vi "Симулятор 1553 windows.vi"() -> ()   [LabVIEW 2015]
panel:
  in  "Управление \nамплитудой, В":dbl(knob)=18.0 min=18.0 max=27.0 scale=18.0..27.0
  out "осталось слов для передачи":u8=1
  out "Режимы машины состояний ОУ":T1=enum."ожидание rising"
  out "Машина состояний КШ":T2
  out "Осталось принять слов":u8=1
  out "Принимаемые\nданные":u16[](array[numeric]) format="%04x"
  out "Передача?":bool=TRUE
  out "Ошибка \nпередачи на ОУ":bool
  out "Подадрес":u32
  out "Передача данных\n на ОУ?":bool
  out "Кол-во СД":u8
  in  "адрес этого\nОУ (0-30)":u8=8
  out "записаны данные":dbl
  out "Waveform Chart":T3(graph)
  out "счетчик длительн бита":u32
  out "T-F crossing":bool
  out "F-T crossing":bool
  in  "Кол-во слов \nдля приема":u8=4
  out "Ошибка \nчтения из ОУ":bool
  in  "RX":bool
  out "TX":bool
  in  "Команда управления":T4(ring)=enum."Блокировать передатчик"
  in  "Отправить команду ОУ":bool
  out "Данные при-\nнятые от КШ":u16[](array[numeric]) format="%04x"
  in  "Данные для\nотправки на КШ":u16[](array[numeric])=[12, 9, 11, 4, 5, 6, 7, 8, 9, 10, 11, 12, 13, 14, 15, 16, 17, 18, 19, 20, 21, 22, 23, 24, 25, 26, 27, 28, 29, 30, 31, 32] format="%04x"
  in  "Отправить\nTx CMD":bool
  in  "Отправить\nRx CMD":bool
  in  "Кол-во слов \nдля передачи":u8=3
  in  "Подадрес (1-30)":u8=1
  in  "адрес ОУ (0-30)":u8=8
  in  "Передаваемые данные":u16[](array[numeric])=[4, 821, 65535, 13380, 0, 0, 0, 0, 0, 0, 0, 0, 0, 0, 0, 0, 0, 0, 0, 0, 0, 0, 0, 0, 0, 0, 0, 0, 0, 0, 0, 0, 0, 0] format="%04x"
  # "Тестовая панель контроллера шины  MIL STD 1553"
  # "Настройки"
  # "Команда передачи:"
  # "Управление ОУ:"
  # "Команда чтения:"
  # "Тестовая панель оконечного устройства шины  MIL STD 1553"
  # "Прием КС:"
  # "Получение:"
  # "Передача:"
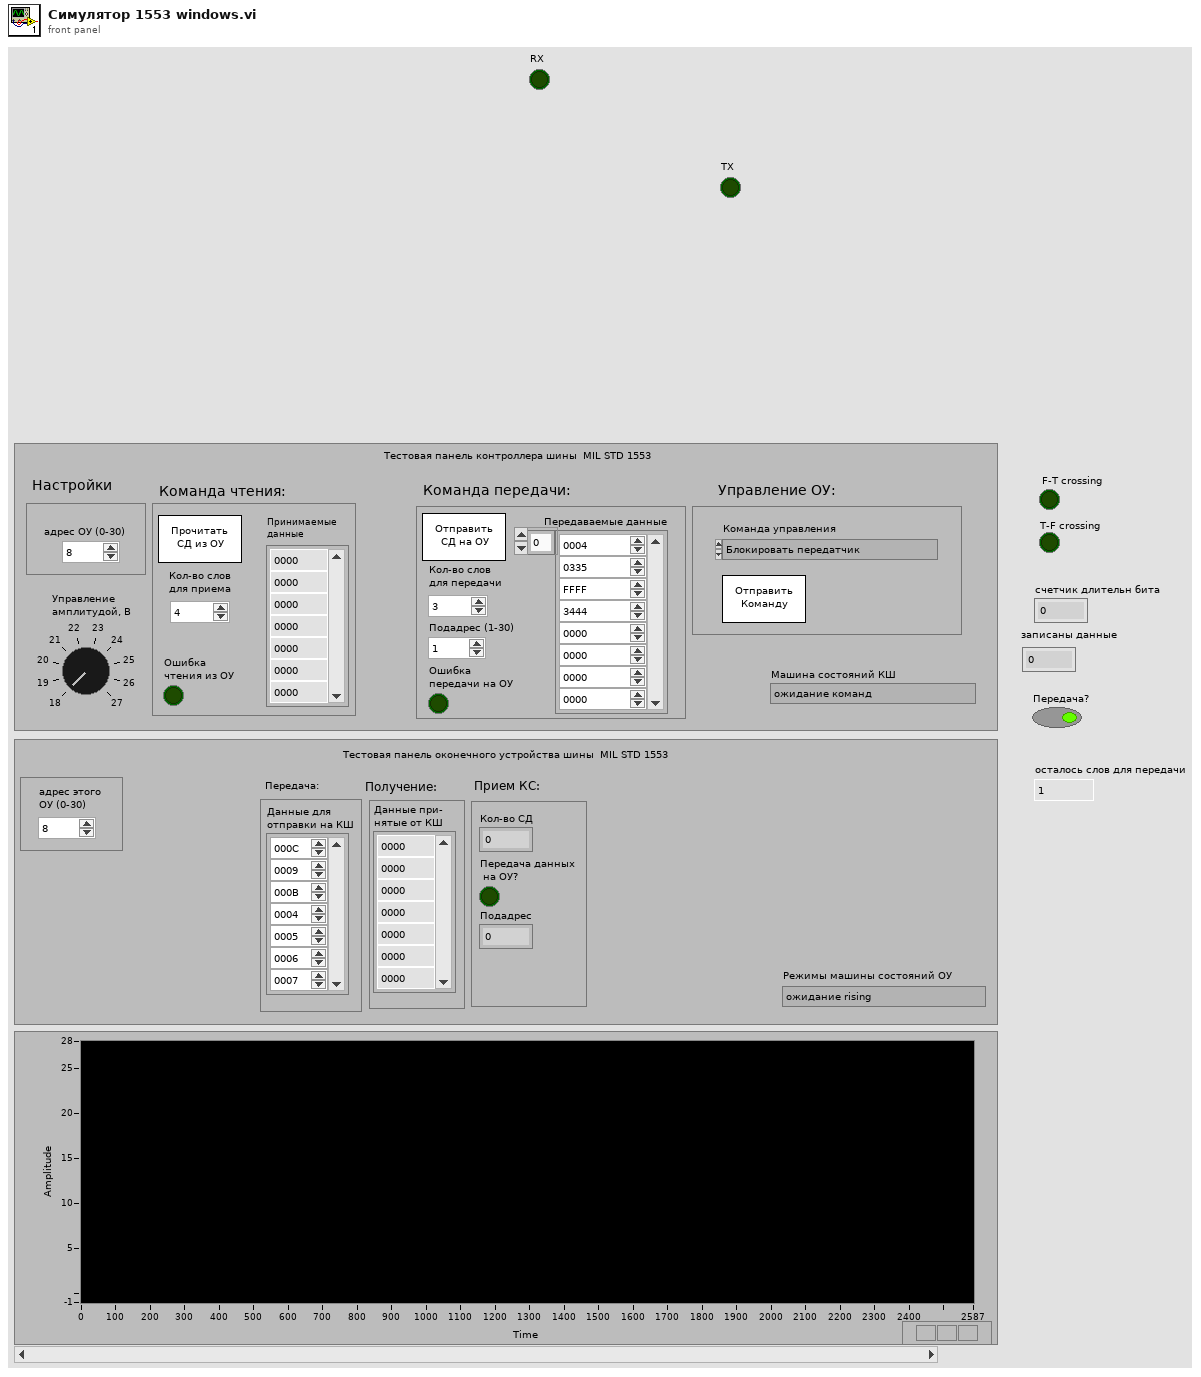
[diagram p1: front panel]
types:
  T1 = typedef "машина состояний ОУ.ctl" = enum16{"замер длительности true", "отправка СД", "кодирование СД", "ожидание rising", "ожидание rising СД", "чтение СД", "чтение КС", "замер длительности true СД", "замер длительности false", "чтение бит КС", "манчестер декодер СД", "манчестер декодер", "чтение бит СД", "подготовка ОС", "кодирование ОС", "отправка ОС", "подготовка СД"}
  T2 = typedef "машина состояний КШ.ctl" = enum16{"ожидание команд", "Подготовка команды RX", "Подготовка команды TX", "кодер манчестер КС", "таймаут t2 между словами", "Передача", "ожидание rising СД", "замер длительности true СД", "чтение бит СД", "манчестер декодер СД", "чтение СД", "ожидание rising ОС", "замер длительности false ОС", "замер длительности true OC", "чтение бит ОС", "манчестер декодер ОС", "чтение ОС", "подготовка СД", "кодирование СД", "отправка СД"}
  T3 = cluster{i16, dbl, "f":dbl, dbl, "записаны данные":dbl}
  T4 = enum16{"Принять управление интерфейсом", "Синхронизация", "Передать ОС", "Начать самоконтроль ОУ", "Блокировать передатчик", "Разблокировать передатчик", "Блокировать признак неисправности ОУ", "Разблокировать признак неисправнотси ОУ", "Установить ОУ в исходное состояние", "Резерв", "Передать векорное слово", "Синхронизвция с СД", "Передать последнюю команду", "Передать слово ВСК ОУ", "Блокировать i-й передатчик", "Разблокировать i-й передатчик", "Резерв 2"}
  T5 = cluster{i16, "f":dbl, "f":dbl, dbl, "записаны данные":dbl}
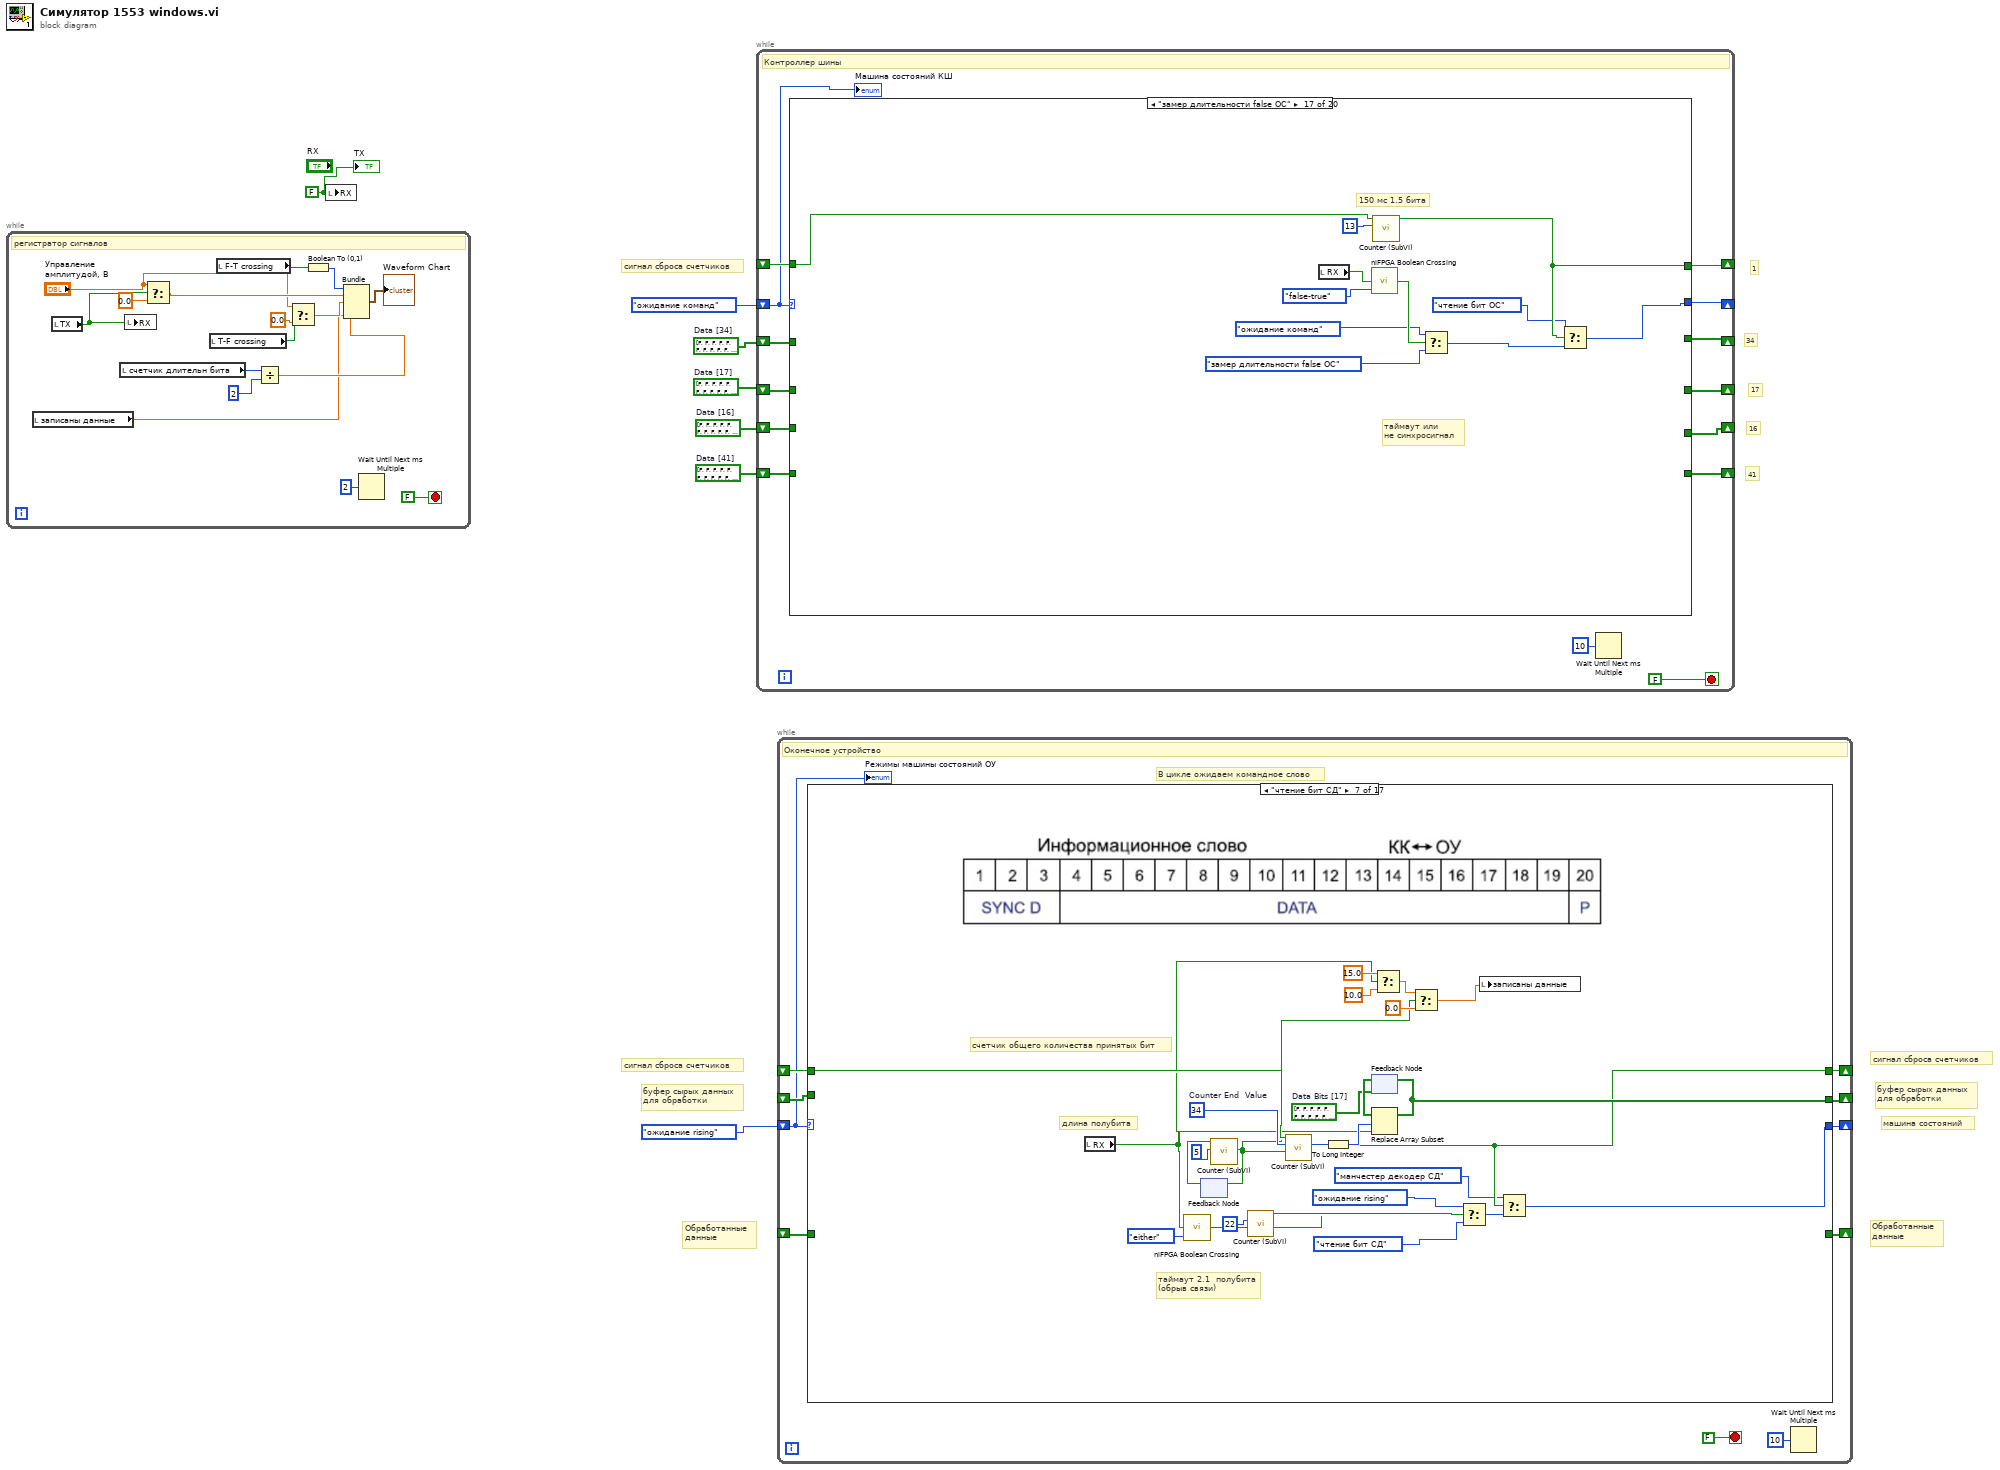
[diagram p0: block diagram]
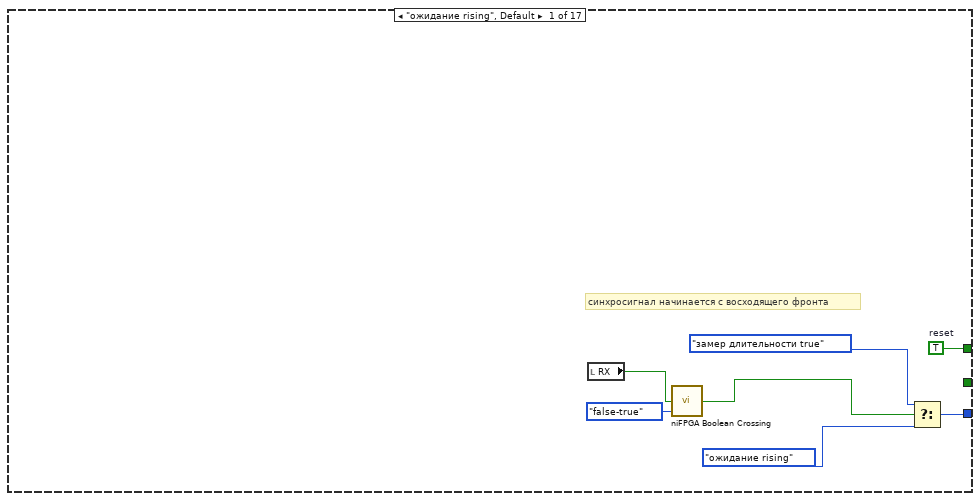
[diagram p2: hidden frame]
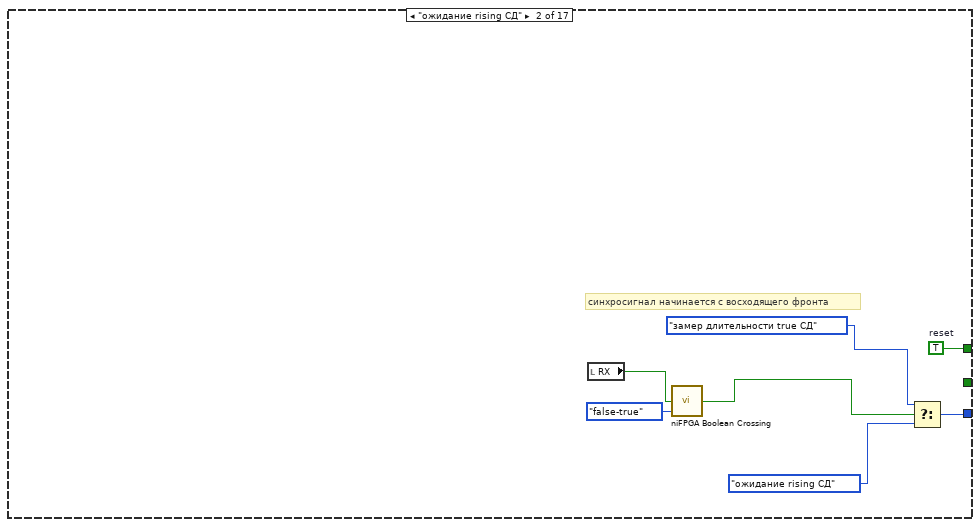
[diagram p3: hidden frame]
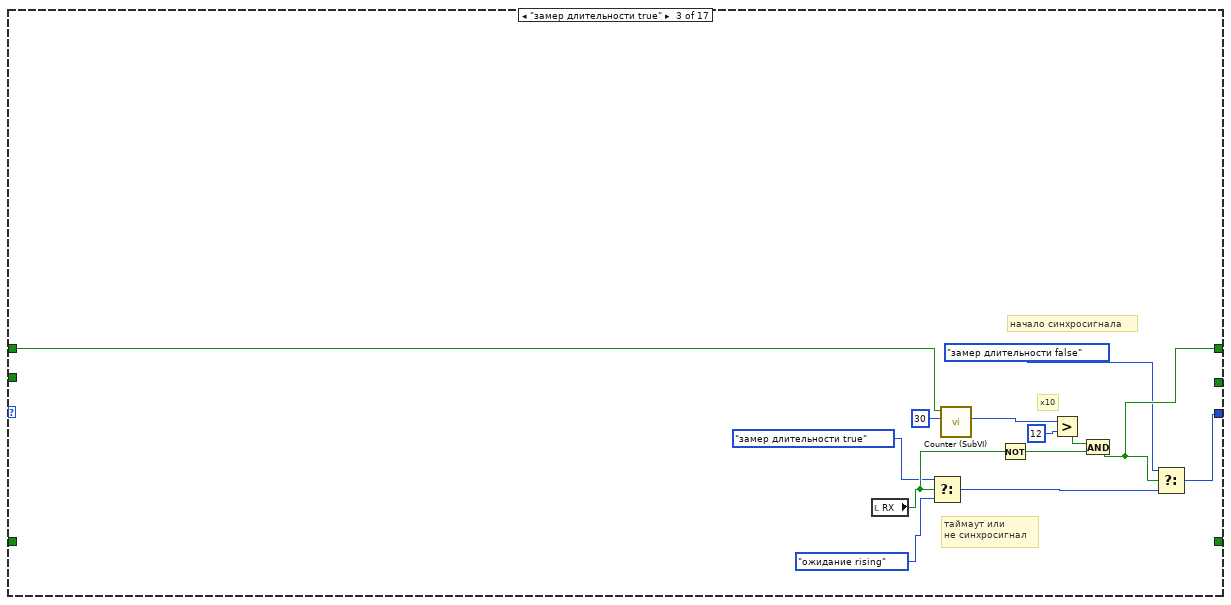
[diagram p4: hidden frame]
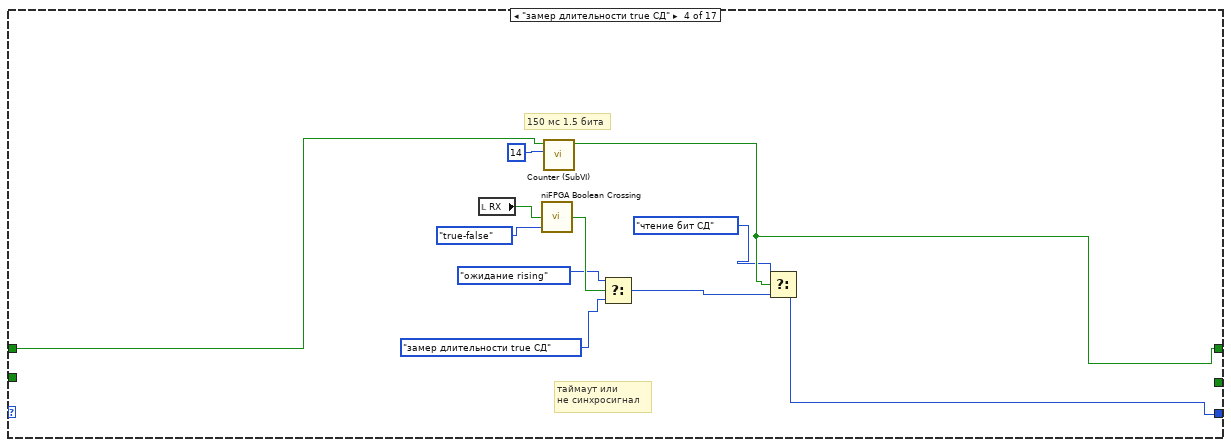
[diagram p5: hidden frame]
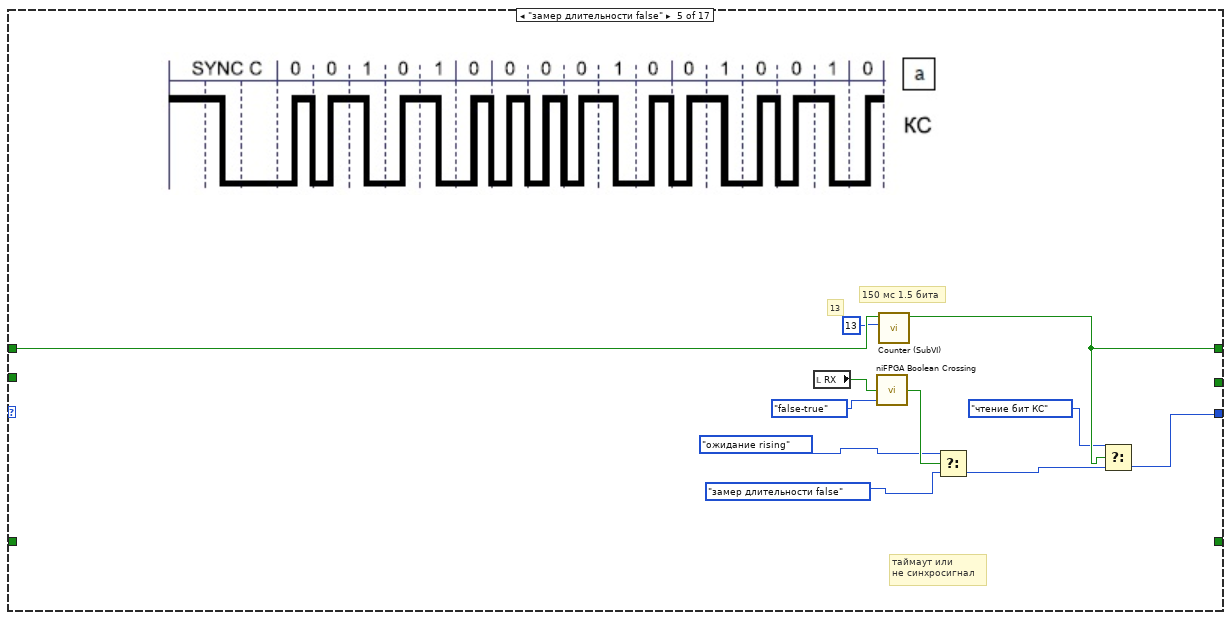
[diagram p6: hidden frame]
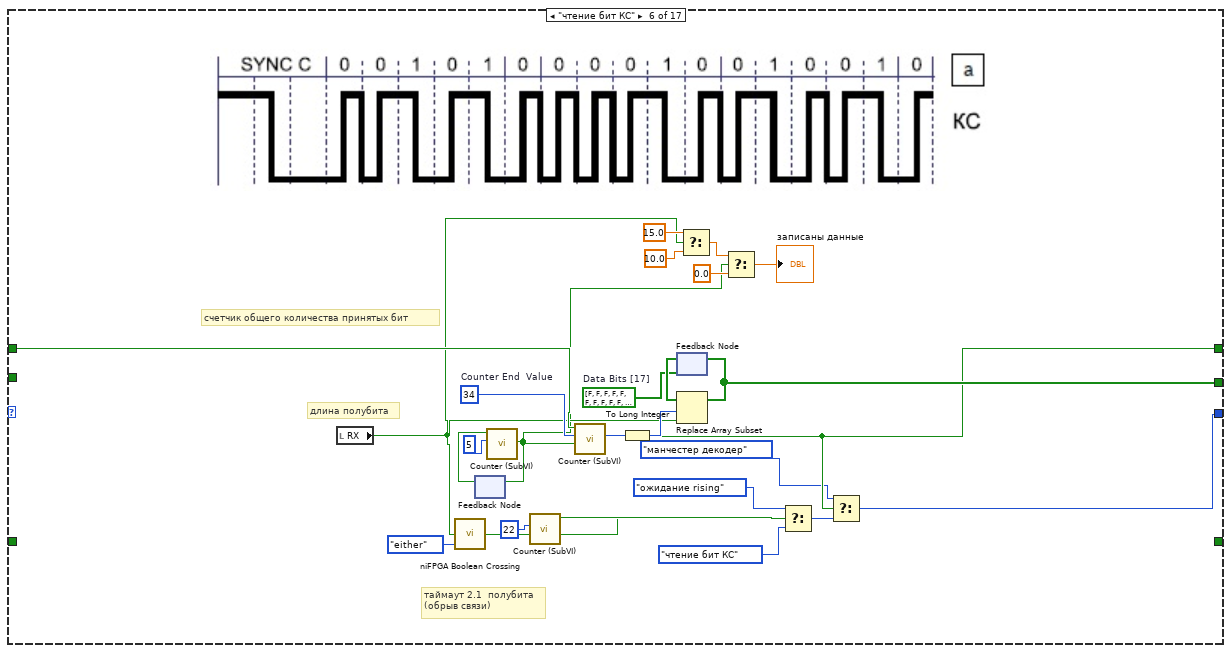
[diagram p7: hidden frame]
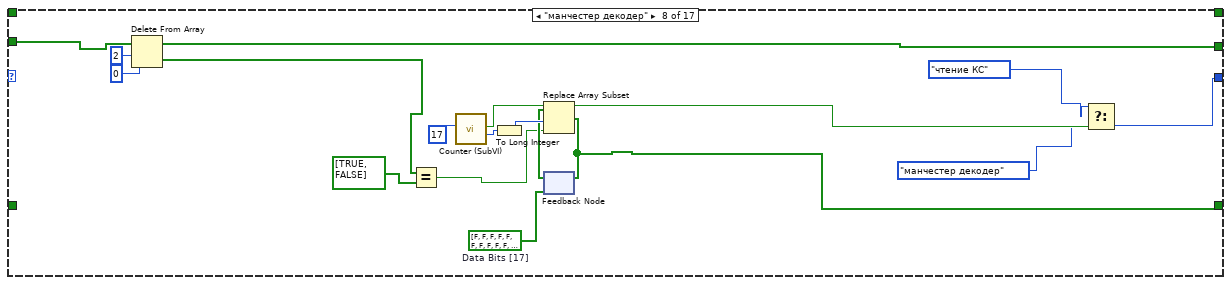
[diagram p8: hidden frame]
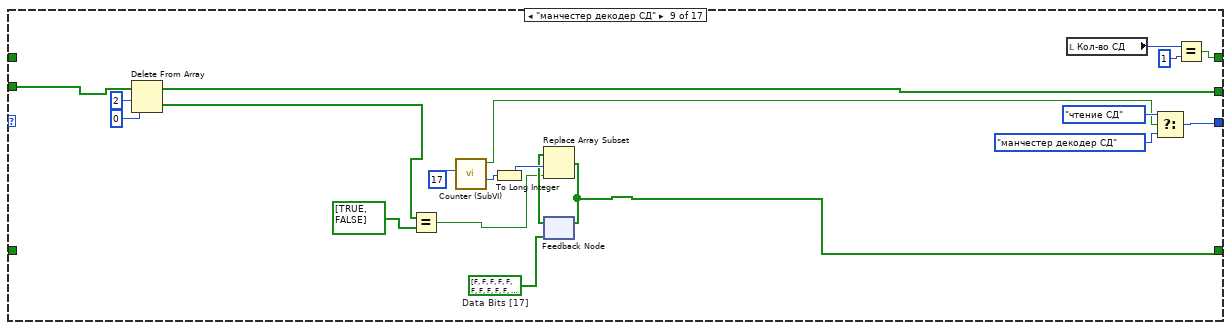
[diagram p9: hidden frame]
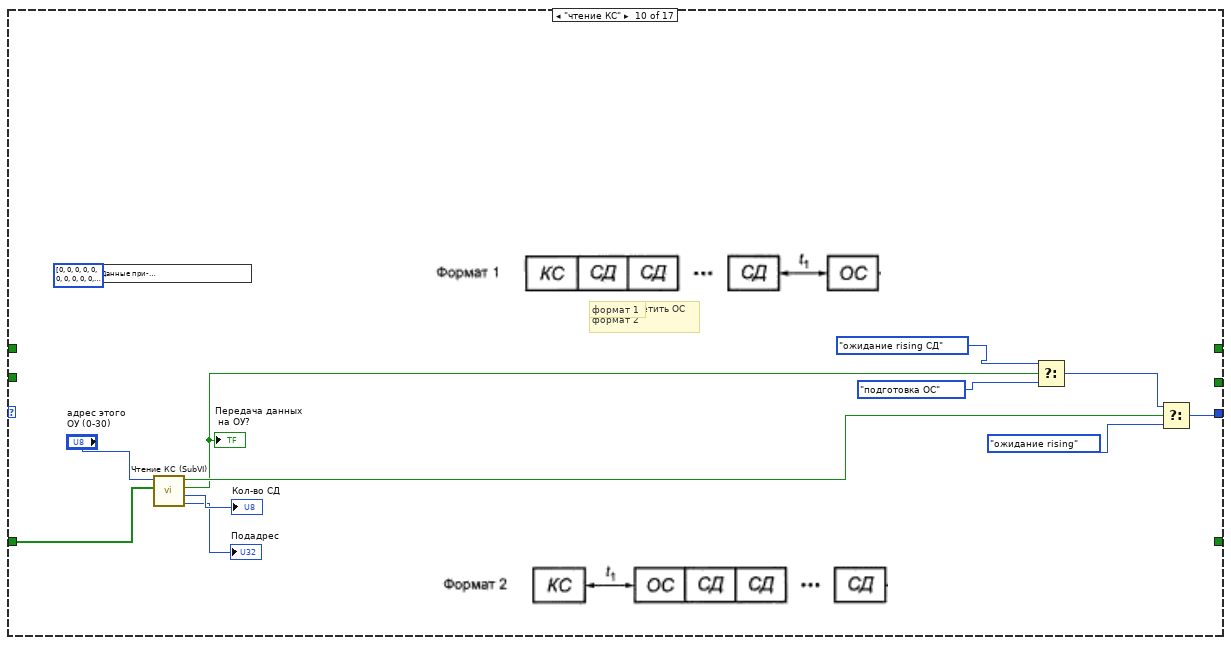
[diagram p10: hidden frame]
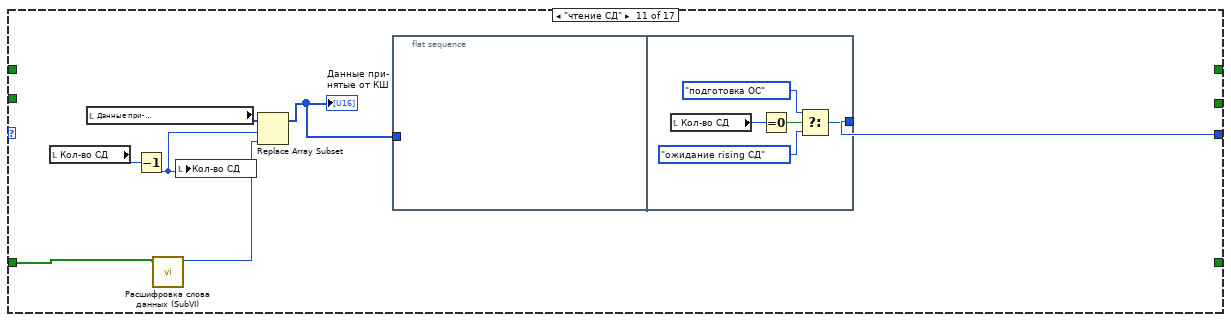
[diagram p11: hidden frame]
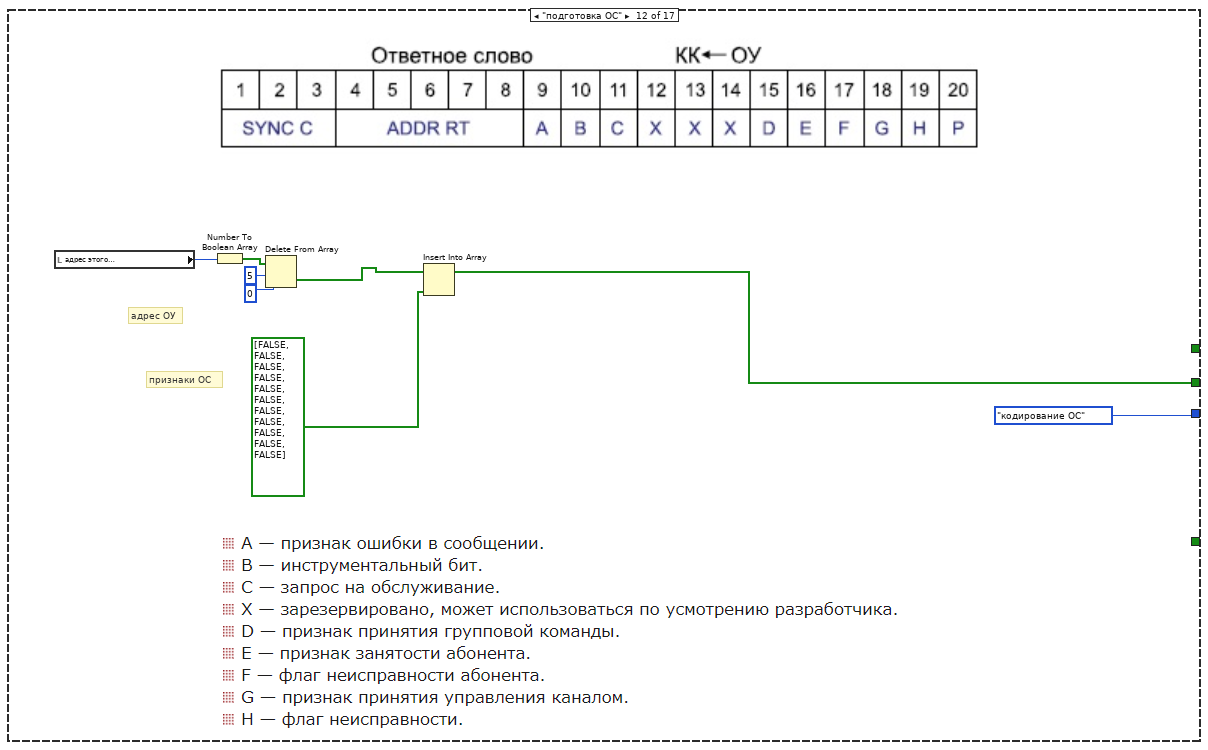
[diagram p12: hidden frame]
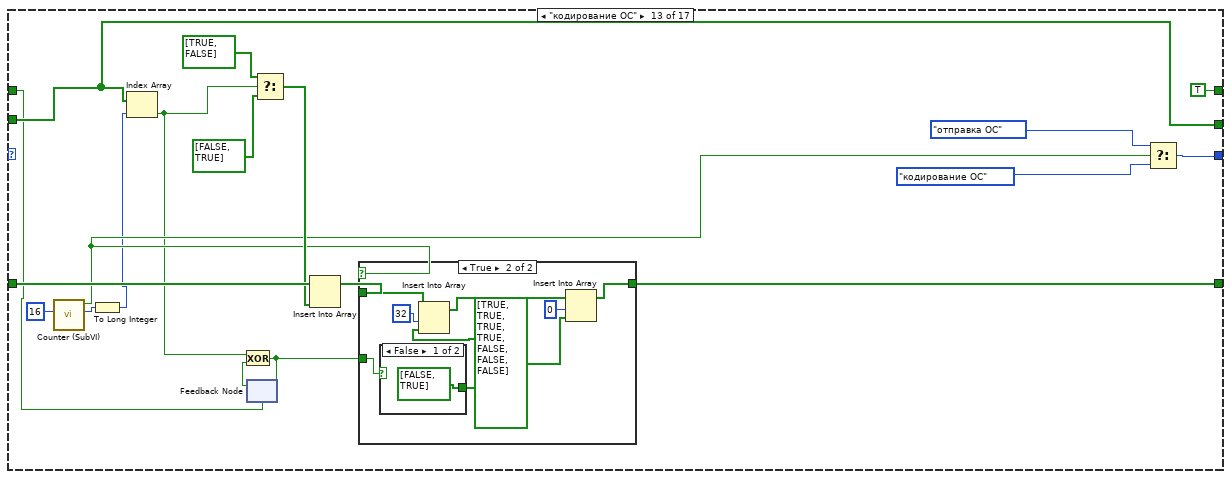
[diagram p13: hidden frame]
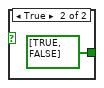
[diagram p15: hidden frame]
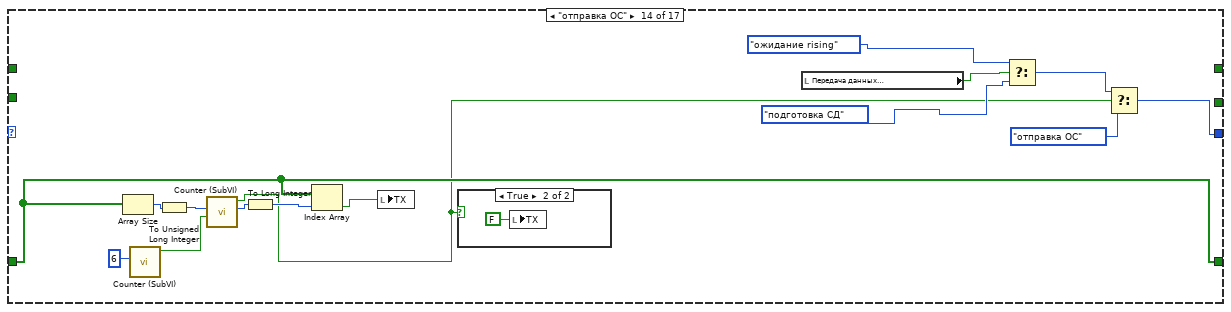
[diagram p16: hidden frame]
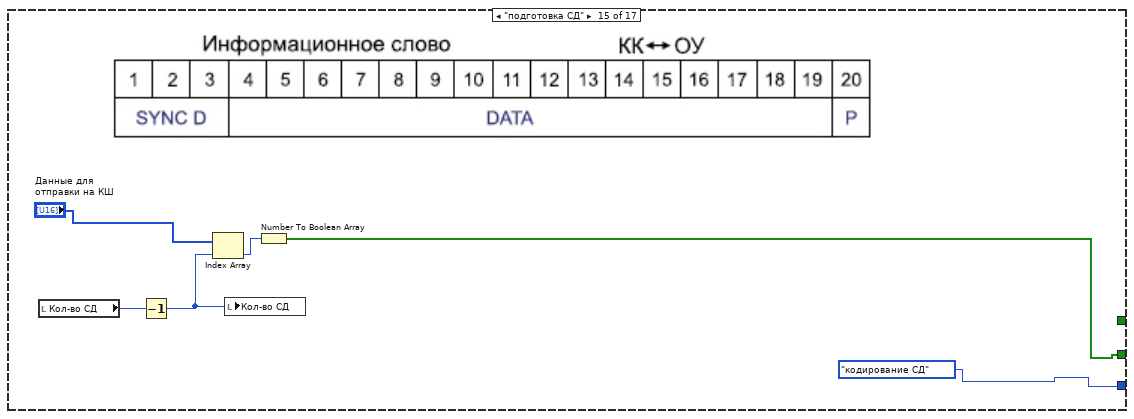
[diagram p18: hidden frame]
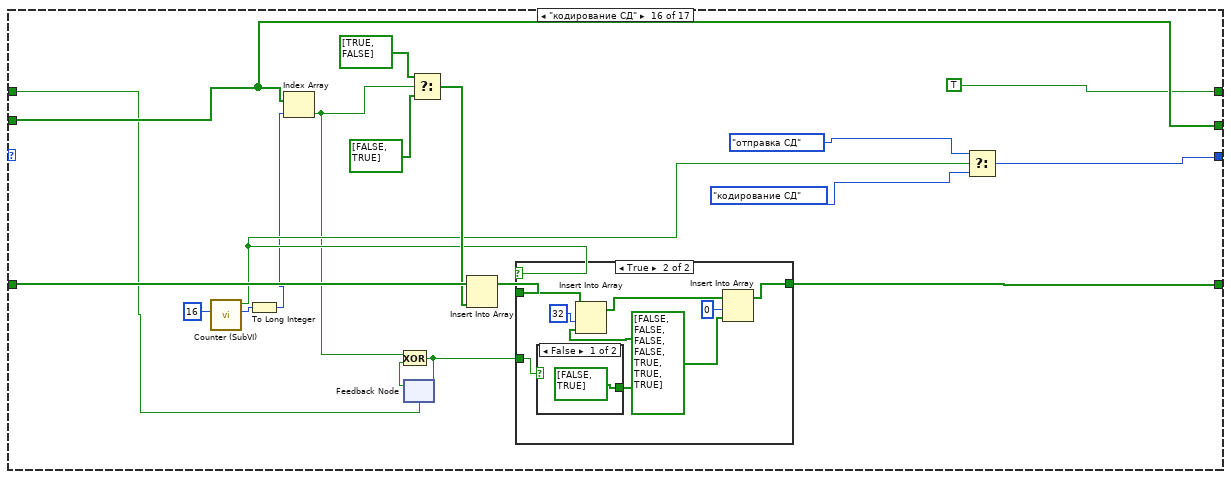
[diagram p19: hidden frame]
diagram:
  w1 = bool[] [FALSE, FALSE, FALSE, FALSE, FALSE, FALSE, FALSE, FALSE, FALSE, FALSE, FALSE, FALSE, FALSE, FALSE, FALSE, FALSE, FALSE, FALSE, FALSE, FALSE, FALSE, FALSE, FALSE, FALSE, FALSE, FALSE, FALSE, FALSE, FALSE, FALSE, FALSE, FALSE, FALSE, FALSE, FALSE, FALSE, FALSE, FALSE, FALSE, FALSE, FALSE]  # Data [41]
  w2 = bool[] [FALSE, FALSE, FALSE, FALSE, FALSE, FALSE, FALSE, FALSE, FALSE, FALSE, FALSE, FALSE, FALSE, FALSE, FALSE, FALSE]  # Data [16]
  w3 = bool[] [FALSE, FALSE, FALSE, FALSE, FALSE, FALSE, FALSE, FALSE, FALSE, FALSE, FALSE, FALSE, FALSE, FALSE, FALSE, FALSE, FALSE]  # Data [17]
  w4 = bool[] [FALSE, FALSE, FALSE, FALSE, FALSE, FALSE, FALSE, FALSE, FALSE, FALSE, FALSE, FALSE, FALSE, FALSE, FALSE, FALSE, FALSE, FALSE, FALSE, FALSE, FALSE, FALSE, FALSE, FALSE, FALSE, FALSE, FALSE, FALSE, FALSE, FALSE, FALSE, FALSE, FALSE, FALSE]  # Data [34]
  w7 = FALSE ("RX")
  # "1"
  # "34"
  # "41"
  # "17"
  # "16"
  # "сигнал сброса счетчиков"
  # "Обработанные\nданные"
  # "буфер сырых данных\nдля обработки"
  # "сигнал сброса счетчиков"
  # "Обработанные\nданные"
  # "машина состояний"
  # "буфер сырых данных\nдля обработки"
  # "сигнал сброса счетчиков"
  n1 = while {
    stop <- FALSE stop-if-true
    # "регистратор сигналов"
    n2 = local read "записаны данные"() -> (w13:dbl)
    n3 = local read "TX"() -> (w10:bool)
    n4 = local read "счетчик длительн бита"() -> (w16:u32)
    n5 = local write "RX"(w10) -> ()
    n6 = Select(t="Управление \nамплитудой, В", s=w10, f=0.0) -> (s? t:f=w11:dbl)
    n7 = local read "T-F crossing"() -> (w19:bool)
    n8 = local read "F-T crossing"() -> (w21:bool)
    n9 = Divide(x=w16, y=u32 2) -> (x/y=w14:dbl)
    n10 = Select(t="Управление \nамплитудой, В", s=w19, f=0.0) -> (s? t:f=w17:dbl)
    n11 = Boolean To (0,1)(Boolean=w21) -> (0, 1=w20:i16)
    n12 = Bundle(w20, "f"=w11, "f"=w17, w14, "записаны данные"=w13) -> (→"Waveform Chart":T5)  [unwired: 1 in]
    n13 = Wait Until Next ms Multiple(millisecond multiple=u32 2) -> ()  [unwired: 1 out]
  }
  n14 = local write "RX"(w7) -> ()
  n15 = while {
    shift-right: [w36] -> _
    shift-left: машина_состояний_КШ."ожидание команд" ("Машина состояний КШ") -> [w24]
    shift-right: [w35] -> _
    shift-left: _ -> [w34]
    shift-right: [w33] -> _
    shift-left: w4 -> [w32]
    shift-right: [w31] -> _
    shift-left: w3 -> [w30]
    shift-right: [w25] -> _
    shift-left: w2 -> [w27]
    shift-right: [w26] -> _
    shift-left: w1 -> [w28]
    stop <- FALSE stop-if-true
    # "Контроллер шины"
    n16 = case shown="\"замер длительности false ОС\"" w24 {
      tunnel: [w45 машина_состояний_КШ."кодер манчестер КС" ("Машина состояний КШ") машина_состояний_КШ."кодер манчестер КС" ("Машина состояний КШ") w85 w115 w126 машина_состояний_КШ."кодирование СД" ("Машина состояний КШ") w150 w175 w199 w209 w220 w230 w244 w276 w292 w302 w312 w347 w360] -> w36
      tunnel: [_ TRUE ("End Reached") TRUE ("End Reached") w82 w107 w122 TRUE ("End Reached") w138 w174 w192 w205 w219 w231 w245 _ _ w301 w315 _ _] -> w35
      tunnel: w34 -> [_ _ _ w72 _ w123 _ w140 _ w190 w206 w221 w232 w243 w264 _ w303 w316 w337 _]
      tunnel: [_ _ _ _ _ _ _ _ _ _ _ _ _ w242 w270 _ _ w313 w336 _] -> w33
      tunnel: w32 -> [_ _ _ _ _ _ _ _ _ _ _ _ _ _ w270 _ _ _ w336 _]
      tunnel: [_ _ _ _ _ _ _ _ _ _ _ _ _ _ w275 _ _ _ w346 _] -> w31
      tunnel: w30 -> [_ _ _ _ _ _ _ _ _ _ _ _ _ _ _ w287 _ _ _ w362]
      tunnel: w28 -> [_ _ _ w69 w106 _ _ w137 w173 _ _ _ _ _ _ _ _ _ _ _]
      tunnel: w27 -> [_ _ _ w68 _ _ _ w135 _ _ _ _ _ _ _ _ _ _ _ _]
      tunnel: [_ _ _ w70 w106 _ _ w136 w173 _ _ _ _ _ _ _ _ _ _ _] -> w26
      tunnel: [_ w47 w57 w68 _ _ w128 w135 _ _ _ _ _ _ _ _ _ _ _ _] -> w25
      frame "ожидание команд", Default {
        # "структура обрабатывает нажатие кнопок \nприема и передачи. При соответствующем нажатии\nмашина состояний переключается  в необходимое состояние"
        # "КШ ожидает приема команды для передачи информации"
        n17 = Or(x="Отправить команду ОУ", y="Отправить\nTx CMD") -> (x .or. y?=w41:bool)
        n18 = Select(t=машина_состояний_КШ."Подготовка команды RX" ("Машина состояний КШ"), s="Отправить\nRx CMD", f=машина_состояний_КШ."ожидание команд" ("Машина состояний КШ")) -> (s? t:f=w44:T2)
        n19 = Select(t=машина_состояний_КШ."Подготовка команды TX" ("Машина состояний КШ"), s=w41, f=w44) -> (s? t:f=w45:T2)
      }
      frame "Подготовка команды TX" {
        w50 = TRUE ("Разряд прием\\передача")
        # "16"
        # "устанавливаем флаг\nпередачи СД от КШ"
        # "следующая операция:\nзакодировать КС\nв манчестер-2"
        # "переменная для хранения\nколичестов СД"
        # "1"
        # "подготавливаем пакет командного слова:"
        n20 = local read "Отправить команду ОУ"() -> (w51:bool)
        n21 = call "Командное слово (SubVI).vi"("Признак команды"=w51, "Кол-во слов (1-32)"="Кол-во слов \nдля передачи", "Команда управления"="Команда управления", "Подадрес (1-30)"="Подадрес (1-30)", "Разряд прием\\передача"=w50, "адрес ОУ (0-30)"="адрес ОУ (0-30)") -> ("КС"=w47:bool[])  [unwired: 5 in]
        n22 = flat-sequence {
          tunnel: w51 -> [_]
          frame #0 {
            n23 = local write "Отправить команду ОУ"(FALSE ("Отправить команду ОУ")) -> ()
          }
        }
        "Передача?" <- w50
        "осталось слов для передачи" <- "Кол-во слов \nдля передачи"
      }
      frame "Подготовка команды RX" {
        w61 = FALSE ("Разряд прием\\передача 2")
        # "16"
        # "следующая операция:\nзакодировать КС\nв манчестер-2"
        # "обнуляем массив входящих данных"
        # "подготавливаем КС,\nвключаем адрем ОУ,\nбит передачи, подадрес\nи число СД"
        n24 = local read "Отправить команду ОУ"() -> (w63:bool)
        n25 = local read "Команда управления"() -> (w64:T4)
        n26 = local read "Подадрес (1-30)"() -> (w65:u8)
        n27 = local read "адрес ОУ (0-30)"() -> (w66:u8)
        n28 = local write "Передача?"(w61) -> ()
        n29 = local write "Принимаемые\nданные"(u16[] []) -> ()
        n30 = call "Командное слово (SubVI).vi"("Признак команды"=w63, "Кол-во слов (1-32)"="Кол-во слов \nдля приема", "Команда управления"=w64, "Подадрес (1-30)"=w65, "Разряд прием\\передача"=w61, "адрес ОУ (0-30)"=w66) -> ("КС"=w57:bool[])  [unwired: 5 in]
        n31 = flat-sequence {
          tunnel: w63 -> [_]
          frame #0 {
            n32 = local write "Отправить команду ОУ"(FALSE ("Отправить команду ОУ")) -> ()
          }
        }
        "Осталось принять слов" <- "Кол-во слов \nдля приема"
      }
      frame "кодер манчестер КС" {
        # "16"
        # "41"
        # "41"
        # "16"
        # "расчет бита четности"
        # "счетчик для подсчета\nколичества кодируемых бит.\nкогда достигнет 16, значит\nсообщение закодировано \nполностью"
        n33 = call "Counter (SubVI).vi"("Counter End  Value"=u32 16) -> ("Counter Value"=w88:u32, "End Reached"=w82:bool)  [unwired: 9 in]
        n34 = To Long Integer(number=w88) -> (32bit integer=w91:i32)
        n35 = Index Array(array=w68, index=w91) -> (element=w93:bool)
        n36 = feedback #1() -> (w74:i32)  [unwired: 1 in]
        n37 = Select(t=7 ("length"), s=w72, f=w74) -> (s? t:f=w71:i32)
        n38 = feedback #2() -> (w92:bool)  [unwired: 1 in]
        n39 = Exclusive Or(1:w92, 2:w93) -> (0:w94:bool)
        n40 = feedback-in #2(w94) -> ()
        n41 = Select(t=bool[] [TRUE, FALSE], s=w93, f=bool[] [FALSE, TRUE]) -> (s? t:f=w77:bool[])
        n42 = Add(x=w71, y=2 ("length")) -> (x+y=w75:i32)
        n43 = feedback-in #1(w75) -> ()
        n44 = Replace Array Subset(array=w69, new element=w77, index=w71) -> (w90:bool[])
        n45 = case shown="True" w82 {
          tunnel: w90 -> [w95 w101]
          tunnel: [w95 w102] -> w79
          tunnel: w94 -> [_ w98]
          frame False {
          }
          frame True {
            n46 = case shown="False" w98 {
              tunnel: [bool[] [FALSE, TRUE] bool[] [TRUE, FALSE]] -> w97
              frame False {
              }
              frame True {
              }
            }
            n47 = Replace Array Subset(array=w101, new element=w97, index=39) -> (w100:bool[])
            n48 = Replace Array Subset(array=w100, new element=bool[] [TRUE, TRUE, TRUE, TRUE, FALSE, FALSE, FALSE], index=0) -> (w102:bool[])
          }
        }
        n49 = feedback #3(bool[] [FALSE, FALSE, FALSE, FALSE, FALSE, FALSE, FALSE, FALSE, FALSE, FALSE, FALSE, FALSE, FALSE, FALSE, FALSE, FALSE, FALSE, FALSE, FALSE, FALSE, FALSE, FALSE, FALSE, FALSE, FALSE, FALSE, FALSE, FALSE, FALSE, FALSE, FALSE, FALSE, FALSE, FALSE, FALSE, FALSE, FALSE, FALSE, FALSE, FALSE, FALSE]) -> (w81:bool[])
        n50 = Replace Array Subset(array=w81, new element=w79, index=0) -> (w70:bool[])
        n51 = feedback-in #3(w70) -> ()
        n52 = Select(t=машина_состояний_КШ."Передача" ("Машина состояний КШ"), s=w82, f=машина_состояний_КШ."кодер манчестер КС" ("Машина состояний КШ")) -> (s? t:f=w85:T2)
      }
      frame "Передача" {
        # "41"
        # "41"
        n53 = Array Size(array=w106) -> (size(s)=w113:i32)
        n54 = call "Counter (SubVI).vi"("Counter End  Value"=u32 6) -> ("End Reached"=w116:bool)  [unwired: 9 in, 1 out]
        n55 = To Unsigned Long Integer(number=w113) -> (unsigned 32bit integer=w112:u32)
        n56 = call "Counter (SubVI).vi"("Input Valid"=w116, "Counter End  Value"=w112) -> ("Counter Value"=w120:u32, "End Reached"=w107:bool)  [unwired: 8 in]
        n57 = To Long Integer(number=w120) -> (32bit integer=w118:i32)
        n58 = Index Array(array=w106, index=w118) -> (element=w119:bool)
        n59 = local write "TX"(w119) -> ()
        n60 = case shown="True" w107 {
          frame False {
          }
          frame True {
            n61 = local write "TX"(FALSE ("TX")) -> ()
          }
        }
        n62 = local read "Передача?"() -> (w109:bool)
        n63 = Select(t=машина_состояний_КШ."подготовка СД" ("Машина состояний КШ"), s=w109, f=машина_состояний_КШ."таймаут t2 между словами" ("Машина состояний КШ")) -> (s? t:f=w110:T2)
        n64 = Select(t=w110, s=w107, f=машина_состояний_КШ."Передача" ("Машина состояний КШ")) -> (s? t:f=w115:T2)
      }
      frame "таймаут t2 между словами" {
        n65 = call "Counter (SubVI).vi"("Counter End  Value"=u32 10, "Reset"=w123) -> ("End Reached"=w122:bool)  [unwired: 8 in, 1 out]
        n66 = Select(t=машина_состояний_КШ."ожидание rising ОС" ("Машина состояний КШ"), s=w122, f=машина_состояний_КШ."таймаут t2 между словами" ("Машина состояний КШ")) -> (s? t:f=w126:T2)
      }
      frame "подготовка СД" {
        # "16"
        n67 = local read "осталось слов для передачи"() -> (w131:u8)
        n68 = Decrement(x=w131) -> (x-1=w130:u8)
        n69 = Index Array(array="Передаваемые данные", index=w130) -> (element=w134:u16)
        n70 = local write "осталось слов для передачи"(w130) -> ()
        n71 = Number To Boolean Array(number=w134) -> (Boolean array=w128:bool[])
      }
      frame "кодирование СД" {
        # "16"
        # "41"
        # "41"
        # "16"
        n72 = call "Counter (SubVI).vi"("Counter End  Value"=u32 16) -> ("Counter Value"=w155:u32, "End Reached"=w138:bool)  [unwired: 9 in]
        n73 = To Long Integer(number=w155) -> (32bit integer=w158:i32)
        n74 = Index Array(array=w135, index=w158) -> (element=w160:bool)
        n75 = feedback #4() -> (w159:bool)  [unwired: 1 in]
        n76 = Exclusive Or(1:w159, 2:w160) -> (0:w161:bool)
        n77 = feedback-in #4(w161) -> ()
        n78 = feedback #5() -> (w144:i32)  [unwired: 1 in]
        n79 = Select(t=7 ("length"), s=w140, f=w144) -> (s? t:f=w139:i32)
        n80 = Select(t=bool[] [TRUE, FALSE], s=w160, f=bool[] [FALSE, TRUE]) -> (s? t:f=w145:bool[])
        n81 = Add(x=w139, y=2 ("length")) -> (x+y=w142:i32)
        n82 = feedback-in #5(w142) -> ()
        n83 = Replace Array Subset(array=w137, new element=w145, index=w139) -> (w157:bool[])
        n84 = case shown="True" w138 {
          tunnel: w157 -> [w162 w168]
          tunnel: [w162 w169] -> w146
          tunnel: w161 -> [_ w165]
          frame False {
          }
          frame True {
            n85 = case shown="False" w165 {
              tunnel: [bool[] [FALSE, TRUE] bool[] [TRUE, FALSE]] -> w164
              frame False {
              }
              frame True {
              }
            }
            n86 = Replace Array Subset(array=w168, new element=w164, index=39) -> (w167:bool[])
            n87 = Replace Array Subset(array=w167, new element=bool[] [FALSE, FALSE, FALSE, FALSE, TRUE, TRUE, TRUE], index=0) -> (w169:bool[])
          }
        }
        n88 = feedback #6(bool[] [FALSE, FALSE, FALSE, FALSE, FALSE, FALSE, FALSE, FALSE, FALSE, FALSE, FALSE, FALSE, FALSE, FALSE, FALSE, FALSE, FALSE, FALSE, FALSE, FALSE, FALSE, FALSE, FALSE, FALSE, FALSE, FALSE, FALSE, FALSE, FALSE, FALSE, FALSE, FALSE, FALSE, FALSE, FALSE, FALSE, FALSE, FALSE, FALSE, FALSE, FALSE]) -> (w149:bool[])
        n89 = Replace Array Subset(array=w149, new element=w146, index=0) -> (w136:bool[])
        n90 = feedback-in #6(w136) -> ()
        n91 = Select(t=машина_состояний_КШ."отправка СД" ("Машина состояний КШ"), s=w138, f=машина_состояний_КШ."кодирование СД" ("Машина состояний КШ")) -> (s? t:f=w150:T2)
      }
      frame "отправка СД" {
        # "41"
        # "41"
        n92 = Array Size(array=w173) -> (size(s)=w179:i32)
        n93 = call "Counter (SubVI).vi"("Counter End  Value"=u32 6) -> ("End Reached"=w181:bool)  [unwired: 9 in, 1 out]
        n94 = To Unsigned Long Integer(number=w179) -> (unsigned 32bit integer=w178:u32)
        n95 = call "Counter (SubVI).vi"("Input Valid"=w181, "Counter End  Value"=w178) -> ("Counter Value"=w185:u32, "End Reached"=w177:bool)  [unwired: 8 in]
        n96 = To Long Integer(number=w185) -> (32bit integer=w183:i32)
        n97 = Index Array(array=w173, index=w183) -> (element=w184:bool)
        n98 = local write "TX"(w184) -> ()
        n99 = case shown="True" w177 {
          frame False {
          }
          frame True {
            n100 = local write "TX"(FALSE ("TX")) -> ()
          }
        }
        n101 = local read "осталось слов для передачи"() -> (w188:u8)
        n102 = Equal To 0?(x=w188) -> (x = 0?=w174:bool)
        n103 = Select(t=машина_состояний_КШ."ожидание rising ОС" ("Машина состояний КШ"), s=w174, f=машина_состояний_КШ."подготовка СД" ("Машина состояний КШ")) -> (s? t:f=w176:T2)
        n104 = Select(t=w176, s=w177, f=машина_состояний_КШ."отправка СД" ("Машина состояний КШ")) -> (s? t:f=w175:T2)
      }
      frame "ожидание rising ОС" {
        # "синхросигнал начинается с восходящего фронта"
        n105 = local read "RX"() -> (w201:bool)
        n106 = call "niFPGA Boolean Crossing.vi"("input"=w201, "direction"=enum8{"either", "false-true", "true-false"}."false-true") -> ("crossing"=w192:bool)  [unwired: 7 in]
        "F-T crossing" <- w192
        n107 = call "Counter (SubVI).vi"("Counter End  Value"=u32 50, "Reset"=w190) -> ("Counter Value"=→"счетчик длительн бита":u32, "End Reached"=w196:bool)  [unwired: 8 in]
        n108 = Select(t=машина_состояний_КШ."замер длительности true OC" ("Машина состояний КШ"), s=w192, f=машина_состояний_КШ."ожидание rising ОС" ("Машина состояний КШ")) -> (s? t:f=w197:T2)
        n109 = local write "Ошибка \nпередачи на ОУ"(w196) -> ()
        n110 = Select(t=машина_состояний_КШ."ожидание команд" ("Машина состояний КШ"), s=w196, f=w197) -> (s? t:f=w199:T2)
        n111 = local write "Ошибка \nчтения из ОУ"(w196) -> ()
        "T-F crossing" <- w190
      }
      frame "ожидание rising СД" {
        # "синхросигнал начинается с восходящего фронта"
        n112 = local read "RX"() -> (w212:bool)
        n113 = call "niFPGA Boolean Crossing.vi"("input"=w212, "direction"=enum8{"either", "false-true", "true-false"}."false-true") -> ("crossing"=w213:bool)  [unwired: 7 in]
        n114 = call "Counter (SubVI).vi"("Counter End  Value"=u32 50, "Reset"=w206) -> ("End Reached"=w207:bool)  [unwired: 8 in, 1 out]
        n115 = Not(x=w207) -> (.not. x?=w205:bool)
        n116 = Select(t=машина_состояний_КШ."замер длительности true СД" ("Машина состояний КШ"), s=w213, f=машина_состояний_КШ."ожидание rising СД" ("Машина состояний КШ")) -> (s? t:f=w210:T2)
        n117 = local write "Ошибка \nпередачи на ОУ"(w207) -> ()
        n118 = Select(t=w210, s=w205, f=машина_состояний_КШ."ожидание команд" ("Машина состояний КШ")) -> (s? t:f=w209:T2)
        n119 = local write "Ошибка \nчтения из ОУ"(w207) -> ()
      }
      frame "замер длительности true OC" {
        # "x10"
        # "начало синхросигнала"
        # "таймаут или \nне синхросигнал"
        n120 = local read "RX"() -> (w218:bool)
        n121 = Select(t=машина_состояний_КШ."замер длительности true OC" ("Машина состояний КШ"), s=w218, f=машина_состояний_КШ."ожидание команд" ("Машина состояний КШ")) -> (s? t:f=w224:T2)
        n122 = call "Counter (SubVI).vi"("Counter End  Value"=u32 30, "Reset"=w221) -> ("Counter Value"=w217:u32)  [unwired: 8 in, 1 out]
        n123 = Not(x=w218) -> (.not. x?=w226:bool)
        n124 = Greater?(x=w217, y=u32 11 ("Counter End  Value")) -> (0:w225:bool)
        n125 = And(x=w225, y=w226) -> (x .and. y?=w219:bool)
        n126 = Select(t=машина_состояний_КШ."замер длительности false ОС" ("Машина состояний КШ"), s=w219, f=w224) -> (s? t:f=w220:T2)
      }
      frame "замер длительности true СД" {
        # "150 мс 1.5 бита"
        # "таймаут или \nне синхросигнал"
        n127 = local read "RX"() -> (w235:bool)
        n128 = call "niFPGA Boolean Crossing.vi"("input"=w235, "direction"=enum8{"either", "false-true", "true-false"}."true-false") -> ("crossing"=w237:bool)  [unwired: 7 in]
        n129 = call "Counter (SubVI).vi"("Counter End  Value"=u32 13, "Reset"=w232) -> ("End Reached"=w231:bool)  [unwired: 8 in, 1 out]
        n130 = Select(t=машина_состояний_КШ."ожидание команд" ("Машина состояний КШ"), s=w237, f=машина_состояний_КШ."замер длительности true СД" ("Машина состояний КШ")) -> (s? t:f=w234:T2)
        n131 = Select(t=машина_состояний_КШ."чтение бит СД" ("Машина состояний КШ"), s=w231, f=w234) -> (s? t:f=w230:T2)
      }
      frame "чтение бит СД" {
        w251 = u32 34  # Counter End  Value
        w248 = bool[] [FALSE, FALSE, FALSE, FALSE, FALSE, FALSE, FALSE, FALSE, FALSE, FALSE, FALSE, FALSE, FALSE, FALSE, FALSE, FALSE, FALSE, FALSE, FALSE, FALSE, FALSE, FALSE, FALSE, FALSE, FALSE, FALSE, FALSE, FALSE, FALSE, FALSE, FALSE, FALSE, FALSE, FALSE]  # Data Bits [17]
        # "34"
        # "длина полубита"
        # "счетчик общего количества принятых бит"
        # "таймаут 2.1  полубита\n(обрыв связи)"
        n132 = local read "RX"() -> (w238:bool)
        n133 = call "niFPGA Boolean Crossing.vi"("input"=w238, "direction"=enum8{"either", "false-true", "true-false"}."either") -> ("crossing"=w261:bool)  [unwired: 7 in]
        n134 = feedback #7() -> (w254:bool)  [unwired: 1 in]
        n135 = call "Counter (SubVI).vi"("Counter End  Value"=u32 5, "Reset"=w254) -> ("End Reached"=w262:bool)  [unwired: 8 in, 1 out]
        n136 = feedback-in #7(w262) -> ()
        n137 = call "Counter (SubVI).vi"("Counter End  Value"=u32 22, "Reset"=w261) -> ("End Reached"=w256:bool)  [unwired: 8 in, 1 out]
        n138 = call "Counter (SubVI).vi"("Input Valid"=w262, "Counter End  Value"=w251, "Reset"=w243) -> ("Counter Value"=w250:u32, "End Reached"=w245:bool)  [unwired: 7 in]
        n139 = To Long Integer(number=w250) -> (32bit integer=w246:i32)
        n140 = feedback #8(w248) -> (w247:bool[])
        n141 = Replace Array Subset(array=w247, new element=w238, index=w246) -> (w242:bool[])
        n142 = feedback-in #8(w242) -> ()
        n143 = Select(t=15.0, s=w238, f=10.0 ("t")) -> (s? t:f=w258:dbl)
        n144 = Select(t=w258, s=w262, f=0.0) -> (s? t:f=w263:dbl)
        n145 = Select(t=машина_состояний_КШ."ожидание команд" ("Машина состояний КШ"), s=w256, f=машина_состояний_КШ."чтение бит СД" ("Машина состояний КШ")) -> (s? t:f=w252:T2)
        n146 = local write "записаны данные"(w263) -> ()
        n147 = Select(t=машина_состояний_КШ."манчестер декодер СД" ("Машина состояний КШ"), s=w245, f=w252) -> (s? t:f=w244:T2)
      }
      frame "манчестер декодер СД" {
        w280 = bool[] [FALSE, FALSE, FALSE, FALSE, FALSE, FALSE, FALSE, FALSE, FALSE, FALSE, FALSE, FALSE, FALSE, FALSE, FALSE, FALSE, FALSE]  # Data Bits [17]
        # "34"
        # "34"
        # "17"
        n148 = feedback #9() -> (w266:i32)  [unwired: 1 in]
        n149 = Select(t=0 ("length"), s=w264, f=w266) -> (s? t:f=w267:i32)
        n150 = Add(x=w267, y=2 ("length")) -> (x+y=w268:i32)
        n151 = feedback-in #9(w268) -> ()
        n152 = Array Subset(array=w270, index=w267, length=2) -> (w271:bool[])
        n153 = Equal?(x=w271, y=bool[] [TRUE, FALSE]) -> (x = y?=w282:bool)
        n154 = call "Counter (SubVI).vi"("Counter End  Value"=u32 17) -> ("Counter Value"=w281:u32, "End Reached"=w283:bool)  [unwired: 9 in]
        n155 = To Long Integer(number=w281) -> (32bit integer=w278:i32)
        n156 = feedback #10(w280) -> (w279:bool[])
        n157 = Replace Array Subset(array=w279, new element=w282, index=w278) -> (w275:bool[])
        n158 = feedback-in #10(w275) -> ()
        n159 = Select(t=машина_состояний_КШ."чтение СД" ("Машина состояний КШ"), s=w283, f=машина_состояний_КШ."манчестер декодер СД" ("Машина состояний КШ")) -> (s? t:f=w276:T2)
      }
      frame "чтение СД" {
        # "17?"
        n160 = local read "Осталось принять слов"() -> (w296:u8)
        n161 = local read "Принимаемые\nданные"() -> (w293:u16[])
        n162 = Decrement(x=w296) -> (x-1=w295:u8)
        n163 = Delete From Array(array=w287, length=16, index=0) -> (deleted portion=w285:bool[])  [unwired: 1 out]
        n164 = Boolean Array To Number(Boolean array=w285) -> (number=w286:u32)
        n165 = Replace Array Subset(array=w293, new element=w286, index=w295) -> (→"Принимаемые\nданные":u16[])
        n166 = local write "Осталось принять слов"(w295) -> ()
        n167 = Equal To 0?(x=w295) -> (x = 0?=w297:bool)
        n168 = Select(t=машина_состояний_КШ."ожидание команд" ("Машина состояний КШ"), s=w297, f=машина_состояний_КШ."ожидание rising СД" ("Машина состояний КШ")) -> (s? t:f=w292:T2)
      }
      frame "замер длительности false ОС" {
        # "150 мс 1.5 бита"
        # "таймаут или \nне синхросигнал"
        n169 = local read "RX"() -> (w306:bool)
        n170 = call "niFPGA Boolean Crossing.vi"("input"=w306, "direction"=enum8{"either", "false-true", "true-false"}."false-true") -> ("crossing"=w308:bool)  [unwired: 7 in]
        n171 = call "Counter (SubVI).vi"("Counter End  Value"=u32 13, "Reset"=w303) -> ("End Reached"=w301:bool)  [unwired: 8 in, 1 out]
        n172 = Select(t=машина_состояний_КШ."ожидание команд" ("Машина состояний КШ"), s=w308, f=машина_состояний_КШ."замер длительности false ОС" ("Машина состояний КШ")) -> (s? t:f=w305:T2)
        n173 = Select(t=машина_состояний_КШ."чтение бит ОС" ("Машина состояний КШ"), s=w301, f=w305) -> (s? t:f=w302:T2)
      }
      frame "чтение бит ОС" {
        w322 = u32 34  # Counter End  Value
        w319 = bool[] [FALSE, FALSE, FALSE, FALSE, FALSE, FALSE, FALSE, FALSE, FALSE, FALSE, FALSE, FALSE, FALSE, FALSE, FALSE, FALSE, FALSE, FALSE, FALSE, FALSE, FALSE, FALSE, FALSE, FALSE, FALSE, FALSE, FALSE, FALSE, FALSE, FALSE, FALSE, FALSE, FALSE, FALSE]  # Data Bits [17]
        # "34"
        # "длина полубита"
        # "счетчик общего количества принятых бит"
        # "таймаут 2.1  полубита\n(обрыв связи)"
        n174 = local read "RX"() -> (w333:bool)
        n175 = call "niFPGA Boolean Crossing.vi"("input"=w333, "direction"=enum8{"either", "false-true", "true-false"}."either") -> ("crossing"=w332:bool)  [unwired: 7 in]
        n176 = feedback #11() -> (w325:bool)  [unwired: 1 in]
        n177 = call "Counter (SubVI).vi"("Counter End  Value"=u32 5, "Reset"=w325) -> ("End Reached"=w334:bool)  [unwired: 8 in, 1 out]
        n178 = feedback-in #11(w334) -> ()
        n179 = call "Counter (SubVI).vi"("Counter End  Value"=u32 22, "Reset"=w332) -> ("End Reached"=w327:bool)  [unwired: 8 in, 1 out]
        n180 = call "Counter (SubVI).vi"("Input Valid"=w334, "Counter End  Value"=w322, "Reset"=w316) -> ("Counter Value"=w321:u32, "End Reached"=w315:bool)  [unwired: 7 in]
        n181 = To Long Integer(number=w321) -> (32bit integer=w317:i32)
        n182 = feedback #12(w319) -> (w318:bool[])
        n183 = Replace Array Subset(array=w318, new element=w333, index=w317) -> (w313:bool[])
        n184 = feedback-in #12(w313) -> ()
        n185 = Select(t=15.0, s=w333, f=10.0 ("t")) -> (s? t:f=w329:dbl)
        n186 = Select(t=w329, s=w334, f=0.0) -> (s? t:f=w314:dbl)
        n187 = Select(t=машина_состояний_КШ."ожидание команд" ("Машина состояний КШ"), s=w327, f=машина_состояний_КШ."чтение бит ОС" ("Машина состояний КШ")) -> (s? t:f=w323:T2)
        n188 = local write "записаны данные"(w314) -> ()
        n189 = Select(t=машина_состояний_КШ."манчестер декодер ОС" ("Машина состояний КШ"), s=w315, f=w323) -> (s? t:f=w312:T2)
      }
      frame "манчестер декодер ОС" {
        w351 = bool[] [FALSE, FALSE, FALSE, FALSE, FALSE, FALSE, FALSE, FALSE, FALSE, FALSE, FALSE, FALSE, FALSE, FALSE, FALSE, FALSE, FALSE]  # Data Bits [17]
        # "34"
        # "17"
        # "34"
        n190 = feedback #13() -> (w339:i32)  [unwired: 1 in]
        n191 = Select(t=0 ("length"), s=w337, f=w339) -> (s? t:f=w340:i32)
        n192 = Add(x=w340, y=2 ("length")) -> (x+y=w341:i32)
        n193 = feedback-in #13(w341) -> ()
        n194 = Array Subset(array=w336, index=w340, length=2) -> (w335:bool[])
        n195 = Equal?(x=w335, y=bool[] [TRUE, FALSE]) -> (x = y?=w353:bool)
        n196 = call "Counter (SubVI).vi"("Counter End  Value"=u32 17) -> ("Counter Value"=w352:u32, "End Reached"=w354:bool)  [unwired: 9 in]
        n197 = To Long Integer(number=w352) -> (32bit integer=w349:i32)
        n198 = feedback #14(w351) -> (w350:bool[])
        n199 = Replace Array Subset(array=w350, new element=w353, index=w349) -> (w346:bool[])
        n200 = feedback-in #14(w346) -> ()
        n201 = Select(t=машина_состояний_КШ."чтение ОС" ("Машина состояний КШ"), s=w354, f=машина_состояний_КШ."манчестер декодер ОС" ("Машина состояний КШ")) -> (s? t:f=w347:T2)
      }
      frame "чтение ОС" {
        # "17"
        n202 = local read "адрес ОУ (0-30)"() -> (w361:u8)
        n203 = call "Прием ОС (SubVI).vi"("Адрес ОУ"=w361, "RX Data"=w362) -> ("Ошибка ОС"=→"Ошибка \nпередачи на ОУ" →"Ошибка \nчтения из ОУ":bool)  [unwired: 8 in, 1 out]
        n204 = local read "Передача?"() -> (w359:bool)
        n205 = Select(t=машина_состояний_КШ."ожидание команд" ("Машина состояний КШ"), s=w359, f=машина_состояний_КШ."ожидание rising СД" ("Машина состояний КШ")) -> (s? t:f=w360:T2)
      }
    }
    n206 = Wait Until Next ms Multiple(millisecond multiple=u32 10) -> ()  [unwired: 1 out]
    "Машина состояний КШ" <- w24
  }
  n207 = while {
    shift-right: [w371] -> _
    shift-left: машина_состояний_ОУ."ожидание rising" ("Режимы машины состояний ОУ") -> [w363]
    shift-right: [w369] -> _
    shift-left: _ -> [w368]
    shift-right: [w367] -> _
    shift-left: _ -> [w366]
    shift-right: [w365] -> _
    shift-left: _ -> [w364]
    stop <- FALSE stop-if-true
    # "В цикле ожидаем командное слово"
    # "Оконечное устройство"
    n208 = case shown="\"чтение бит СД\"" w363 {
      tunnel: [w377 w384 w396 w404 w421 w440 w466 w479 w500 w517 w526 машина_состояний_ОУ."кодирование ОС" ("Режимы машины состояний ОУ") w561 w574 машина_состояний_ОУ."кодирование СД" ("Режимы машины состояний ОУ") w613 w629] -> w371
      tunnel: [w375 w382 w390 w403 w419 w425 w452 _ w491 _ _ _ TRUE ("End Reached") _ _ TRUE ("End Reached") _] -> w369
      tunnel: w368 -> [_ _ w392 w405 w420 w437 w463 _ _ _ _ _ w546 _ _ w598 _]
      tunnel: [_ _ _ _ _ w426 w453 w486 w506 _ _ w537 w547 _ w593 w599 _] -> w367
      tunnel: w366 -> [_ _ _ _ _ _ _ w487 w507 _ _ _ w547 _ _ w599 _]
      tunnel: [_ _ _ _ _ _ _ w476 w497 _ _ _ w552 w577 _ w604 _] -> w365
      tunnel: w364 -> [_ _ _ _ _ _ _ _ _ w521 w529 _ w558 w577 _ w610 w630]
      frame "ожидание rising", Default {
        w375 = TRUE  # reset
        # "синхросигнал начинается с восходящего фронта"
        n209 = local read "RX"() -> (w378:bool)
        n210 = call "niFPGA Boolean Crossing.vi"("input"=w378, "direction"=enum8{"either", "false-true", "true-false"}."false-true") -> ("crossing"=w376:bool)  [unwired: 7 in]
        n211 = Select(t=машина_состояний_ОУ."замер длительности true" ("Режимы машины состояний ОУ"), s=w376, f=машина_состояний_ОУ."ожидание rising" ("Режимы машины состояний ОУ")) -> (s? t:f=w377:T1)
      }
      frame "ожидание rising СД" {
        w382 = TRUE  # reset
        # "синхросигнал начинается с восходящего фронта"
        n212 = local read "RX"() -> (w385:bool)
        n213 = call "niFPGA Boolean Crossing.vi"("input"=w385, "direction"=enum8{"either", "false-true", "true-false"}."false-true") -> ("crossing"=w383:bool)  [unwired: 7 in]
        n214 = Select(t=машина_состояний_ОУ."замер длительности true СД" ("Режимы машины состояний ОУ"), s=w383, f=машина_состояний_ОУ."ожидание rising СД" ("Режимы машины состояний ОУ")) -> (s? t:f=w384:T1)
      }
      frame "замер длительности true" {
        # "x10"
        # "начало синхросигнала"
        # "таймаут или \nне синхросигнал"
        n215 = local read "RX"() -> (w394:bool)
        n216 = Select(t=машина_состояний_ОУ."замер длительности true" ("Режимы машины состояний ОУ"), s=w394, f=машина_состояний_ОУ."ожидание rising" ("Режимы машины состояний ОУ")) -> (s? t:f=w397:T1)
        n217 = call "Counter (SubVI).vi"("Counter End  Value"=u32 30, "Reset"=w392) -> ("Counter Value"=w391:u32)  [unwired: 8 in, 1 out]
        n218 = Not(x=w394) -> (.not. x?=w393:bool)
        n219 = Greater?(x=w391, y=u32 12 ("Counter End  Value")) -> (0:w395:bool)
        n220 = And(x=w395, y=w393) -> (x .and. y?=w390:bool)
        n221 = Select(t=машина_состояний_ОУ."замер длительности false" ("Режимы машины состояний ОУ"), s=w390, f=w397) -> (s? t:f=w396:T1)
      }
      frame "замер длительности true СД" {
        # "150 мс 1.5 бита"
        # "таймаут или \nне синхросигнал"
        n222 = local read "RX"() -> (w408:bool)
        n223 = call "niFPGA Boolean Crossing.vi"("input"=w408, "direction"=enum8{"either", "false-true", "true-false"}."true-false") -> ("crossing"=w406:bool)  [unwired: 7 in]
        n224 = call "Counter (SubVI).vi"("Counter End  Value"=u32 14, "Reset"=w405) -> ("End Reached"=w403:bool)  [unwired: 8 in, 1 out]
        n225 = Select(t=машина_состояний_ОУ."ожидание rising" ("Режимы машины состояний ОУ"), s=w406, f=машина_состояний_ОУ."замер длительности true СД" ("Режимы машины состояний ОУ")) -> (s? t:f=w409:T1)
        n226 = Select(t=машина_состояний_ОУ."чтение бит СД" ("Режимы машины состояний ОУ"), s=w403, f=w409) -> (s? t:f=w404:T1)
      }
      frame "замер длительности false" {
        # "13"
        # "150 мс 1.5 бита"
        # "таймаут или \nне синхросигнал"
        n227 = local read "RX"() -> (w416:bool)
        n228 = call "niFPGA Boolean Crossing.vi"("input"=w416, "direction"=enum8{"either", "false-true", "true-false"}."false-true") -> ("crossing"=w414:bool)  [unwired: 7 in]
        n229 = call "Counter (SubVI).vi"("Counter End  Value"=u32 13, "Reset"=w420) -> ("End Reached"=w419:bool)  [unwired: 8 in, 1 out]
        n230 = Select(t=машина_состояний_ОУ."ожидание rising" ("Режимы машины состояний ОУ"), s=w414, f=машина_состояний_ОУ."замер длительности false" ("Режимы машины состояний ОУ")) -> (s? t:f=w417:T1)
        n231 = Select(t=машина_состояний_ОУ."чтение бит КС" ("Режимы машины состояний ОУ"), s=w419, f=w417) -> (s? t:f=w421:T1)
      }
      frame "чтение бит КС" {
        w442 = u32 34  # Counter End  Value
        w445 = bool[] [FALSE, FALSE, FALSE, FALSE, FALSE, FALSE, FALSE, FALSE, FALSE, FALSE, FALSE, FALSE, FALSE, FALSE, FALSE, FALSE, FALSE, FALSE, FALSE, FALSE, FALSE, FALSE, FALSE, FALSE, FALSE, FALSE, FALSE, FALSE, FALSE, FALSE, FALSE, FALSE, FALSE, FALSE]  # Data Bits [17]
        # "длина полубита"
        # "счетчик общего количества принятых бит"
        # "таймаут 2.1  полубита\n(обрыв связи)"
        n232 = local read "RX"() -> (w428:bool)
        n233 = call "niFPGA Boolean Crossing.vi"("input"=w428, "direction"=enum8{"either", "false-true", "true-false"}."either") -> ("crossing"=w429:bool)  [unwired: 7 in]
        n234 = feedback #15() -> (w438:bool)  [unwired: 1 in]
        n235 = call "Counter (SubVI).vi"("Counter End  Value"=u32 5, "Reset"=w438) -> ("End Reached"=w427:bool)  [unwired: 8 in, 1 out]
        n236 = feedback-in #15(w427) -> ()
        n237 = call "Counter (SubVI).vi"("Counter End  Value"=u32 22, "Reset"=w429) -> ("End Reached"=w435:bool)  [unwired: 8 in, 1 out]
        n238 = call "Counter (SubVI).vi"("Input Valid"=w427, "Counter End  Value"=w442, "Reset"=w437) -> ("Counter Value"=w443:u32, "End Reached"=w425:bool)  [unwired: 7 in]
        n239 = To Long Integer(number=w443) -> (32bit integer=w447:i32)
        n240 = feedback #16(w445) -> (w446:bool[])
        n241 = Replace Array Subset(array=w446, new element=w428, index=w447) -> (w426:bool[])
        n242 = feedback-in #16(w426) -> ()
        n243 = Select(t=15.0, s=w428, f=10.0 ("t")) -> (s? t:f=w432:dbl)
        n244 = Select(t=w432, s=w427, f=0.0) -> (s? t:f=→"записаны данные":dbl)
        n245 = Select(t=машина_состояний_ОУ."ожидание rising" ("Режимы машины состояний ОУ"), s=w435, f=машина_состояний_ОУ."чтение бит КС" ("Режимы машины состояний ОУ")) -> (s? t:f=w441:T1)
        n246 = Select(t=машина_состояний_ОУ."манчестер декодер" ("Режимы машины состояний ОУ"), s=w425, f=w441) -> (s? t:f=w440:T1)
      }
      frame "чтение бит СД" {
        w468 = u32 34  # Counter End  Value
        w471 = bool[] [FALSE, FALSE, FALSE, FALSE, FALSE, FALSE, FALSE, FALSE, FALSE, FALSE, FALSE, FALSE, FALSE, FALSE, FALSE, FALSE, FALSE, FALSE, FALSE, FALSE, FALSE, FALSE, FALSE, FALSE, FALSE, FALSE, FALSE, FALSE, FALSE, FALSE, FALSE, FALSE, FALSE, FALSE]  # Data Bits [17]
        # "длина полубита"
        # "счетчик общего количества принятых бит"
        # "таймаут 2.1  полубита\n(обрыв связи)"
        n247 = local read "RX"() -> (w455:bool)
        n248 = call "niFPGA Boolean Crossing.vi"("input"=w455, "direction"=enum8{"either", "false-true", "true-false"}."either") -> ("crossing"=w456:bool)  [unwired: 7 in]
        n249 = feedback #17() -> (w464:bool)  [unwired: 1 in]
        n250 = call "Counter (SubVI).vi"("Counter End  Value"=u32 5, "Reset"=w464) -> ("End Reached"=w454:bool)  [unwired: 8 in, 1 out]
        n251 = feedback-in #17(w454) -> ()
        n252 = call "Counter (SubVI).vi"("Counter End  Value"=u32 22, "Reset"=w456) -> ("End Reached"=w461:bool)  [unwired: 8 in, 1 out]
        n253 = call "Counter (SubVI).vi"("Input Valid"=w454, "Counter End  Value"=w468, "Reset"=w463) -> ("Counter Value"=w469:u32, "End Reached"=w452:bool)  [unwired: 7 in]
        n254 = To Long Integer(number=w469) -> (32bit integer=w473:i32)
        n255 = feedback #18(w471) -> (w472:bool[])
        n256 = Replace Array Subset(array=w472, new element=w455, index=w473) -> (w453:bool[])
        n257 = feedback-in #18(w453) -> ()
        n258 = Select(t=15.0, s=w455, f=10.0 ("t")) -> (s? t:f=w459:dbl)
        n259 = Select(t=w459, s=w454, f=0.0) -> (s? t:f=w451:dbl)
        n260 = Select(t=машина_состояний_ОУ."ожидание rising" ("Режимы машины состояний ОУ"), s=w461, f=машина_состояний_ОУ."чтение бит СД" ("Режимы машины состояний ОУ")) -> (s? t:f=w467:T1)
        n261 = local write "записаны данные"(w451) -> ()
        n262 = Select(t=машина_состояний_ОУ."манчестер декодер СД" ("Режимы машины состояний ОУ"), s=w452, f=w467) -> (s? t:f=w466:T1)
      }
      frame "манчестер декодер" {
        w483 = bool[] [FALSE, FALSE, FALSE, FALSE, FALSE, FALSE, FALSE, FALSE, FALSE, FALSE, FALSE, FALSE, FALSE, FALSE, FALSE, FALSE, FALSE]  # Data Bits [17]
        n263 = Delete From Array(array=w487, length=2, index=0) -> (deleted portion=w488:bool[], array with subset deleted=w486:bool[])
        n264 = Equal?(x=w488, y=bool[] [TRUE, FALSE]) -> (x = y?=w481:bool)
        n265 = call "Counter (SubVI).vi"("Counter End  Value"=u32 17) -> ("Counter Value"=w482:u32, "End Reached"=w480:bool)  [unwired: 9 in]
        n266 = To Long Integer(number=w482) -> (32bit integer=w485:i32)
        n267 = feedback #19(w483) -> (w484:bool[])
        n268 = Replace Array Subset(array=w484, new element=w481, index=w485) -> (w476:bool[])
        n269 = feedback-in #19(w476) -> ()
        n270 = Select(t=машина_состояний_ОУ."чтение КС" ("Режимы машины состояний ОУ"), s=w480, f=машина_состояний_ОУ."манчестер декодер" ("Режимы машины состояний ОУ")) -> (s? t:f=w479:T1)
      }
      frame "манчестер декодер СД" {
        w503 = bool[] [FALSE, FALSE, FALSE, FALSE, FALSE, FALSE, FALSE, FALSE, FALSE, FALSE, FALSE, FALSE, FALSE, FALSE, FALSE, FALSE, FALSE]  # Data Bits [17]
        n271 = Delete From Array(array=w507, length=2, index=0) -> (deleted portion=w508:bool[], array with subset deleted=w506:bool[])
        n272 = Equal?(x=w508, y=bool[] [TRUE, FALSE]) -> (x = y?=w501:bool)
        n273 = call "Counter (SubVI).vi"("Counter End  Value"=u32 17) -> ("Counter Value"=w502:u32, "End Reached"=w494:bool)  [unwired: 9 in]
        n274 = To Long Integer(number=w502) -> (32bit integer=w505:i32)
        n275 = feedback #20(w503) -> (w504:bool[])
        n276 = Replace Array Subset(array=w504, new element=w501, index=w505) -> (w497:bool[])
        n277 = feedback-in #20(w497) -> ()
        n278 = local read "Кол-во СД"() -> (w493:u8)
        n279 = Select(t=машина_состояний_ОУ."чтение СД" ("Режимы машины состояний ОУ"), s=w494, f=машина_состояний_ОУ."манчестер декодер СД" ("Режимы машины состояний ОУ")) -> (s? t:f=w500:T1)
        n280 = Equal?(x=w493, y=u8 1) -> (x = y?=w491:bool)
      }
      frame "чтение КС" {
        # "формат 1"
        # "нужно ответить ОС\nформат 2"
        n281 = local write "Данные при-\nнятые от КШ"(u16[] [0, 0, 0, 0, 0, 0, 0, 0, 0, 0, 0, 0, 0, 0, 0, 0, 0, 0, 0, 0, 0, 0, 0, 0, 0, 0, 0, 0, 0, 0, 0, 0] ("Чтение:")) -> ()
        n282 = call "Чтение КС (SubVI).vi"("КС для обработки"=w521, "Адрес ОУ (0-31)"="адрес этого\nОУ (0-30)") -> ("Подадрес"=→"Подадрес":u32, "Кол-во СД"=→"Кол-во СД":u32, "Передача данных на ОУ?"=w515:bool, "КС верно?"=w518:bool)  [unwired: 6 in]
        "Передача данных\n на ОУ?" <- w515
        n283 = Select(t=машина_состояний_ОУ."ожидание rising СД" ("Режимы машины состояний ОУ"), s=w515, f=машина_состояний_ОУ."подготовка ОС" ("Режимы машины состояний ОУ")) -> (s? t:f=w516:T1)
        n284 = Select(t=w516, s=w518, f=машина_состояний_ОУ."ожидание rising" ("Режимы машины состояний ОУ")) -> (s? t:f=w517:T1)
      }
      frame "чтение СД" {
        n285 = local read "Кол-во СД"() -> (w525:u8)
        n286 = local read "Данные при-\nнятые от КШ"() -> (w528:u16[])
        n287 = Decrement(x=w525) -> (x-1=w524:u8)
        n288 = call "Расшифровка слова данных (SubVI).vi"("СД"=w529) -> ("Data"=w527:u16)  [unwired: 9 in, 1 out]
        n289 = local write "Кол-во СД"(w524) -> ()
        n290 = Replace Array Subset(array=w528, new element=w527, index=w524) -> (w523:u16[])
        "Данные при-\nнятые от КШ" <- w523
        n291 = flat-sequence {
          tunnel: w523 -> [_]
          tunnel: [w534] -> w526
          frame #0 {
          }
          frame #1 {
            n292 = local read "Кол-во СД"() -> (w530:u8)
            n293 = Equal To 0?(x=w530) -> (x = 0?=w533:bool)
            n294 = Select(t=машина_состояний_ОУ."подготовка ОС" ("Режимы машины состояний ОУ"), s=w533, f=машина_состояний_ОУ."ожидание rising СД" ("Режимы машины состояний ОУ")) -> (s? t:f=w534:T1)
          }
        }
      }
      frame "подготовка ОС" {
        # "адрес ОУ"
        # "признаки ОС"
        n295 = local read "адрес этого\nОУ (0-30)"() -> (w542:u8)
        n296 = Number To Boolean Array(number=w542) -> (Boolean array=w541:bool[])
        n297 = Delete From Array(array=w541, length=5, index=0) -> (deleted portion=w536:bool[])  [unwired: 1 out]
        n298 = Insert Into Array(array=w536, new element=bool[] [FALSE, FALSE, FALSE, FALSE, FALSE, FALSE, FALSE, FALSE, FALSE, FALSE, FALSE] ("Признак ОС")) -> (w537:bool[])  [unwired: 1 in]
      }
      frame "кодирование ОС" {
        n299 = call "Counter (SubVI).vi"("Counter End  Value"=u32 16) -> ("Counter Value"=w556:u32, "End Reached"=w554:bool)  [unwired: 9 in]
        n300 = To Long Integer(number=w556) -> (32bit integer=w551:i32)
        n301 = Index Array(array=w547, index=w551) -> (element=w549:bool)
        n302 = feedback #21(w546) -> (w550:bool)
        n303 = Exclusive Or(1:w550, 2:w549) -> (0:w548:bool)
        n304 = feedback-in #21(w548) -> ()
        n305 = Select(t=bool[] [TRUE, FALSE], s=w549, f=bool[] [FALSE, TRUE]) -> (s? t:f=w557:bool[])
        n306 = Insert Into Array(array=w558, new element=w557) -> (w553:bool[])  [unwired: 1 in]
        n307 = case shown="True" w554 {
          tunnel: w553 -> [w562 w568]
          tunnel: [w562 w569] -> w552
          tunnel: w548 -> [_ w565]
          frame False {
          }
          frame True {
            n308 = case shown="False" w565 {
              tunnel: [bool[] [FALSE, TRUE] bool[] [TRUE, FALSE]] -> w564
              frame False {
              }
              frame True {
              }
            }
            n309 = Insert Into Array(array=w568, index=32, new element=w564) -> (w567:bool[])
            n310 = Insert Into Array(array=w567, index=0, new element=bool[] [TRUE, TRUE, TRUE, TRUE, FALSE, FALSE, FALSE]) -> (w569:bool[])
          }
        }
        n311 = Select(t=машина_состояний_ОУ."отправка ОС" ("Режимы машины состояний ОУ"), s=w554, f=машина_состояний_ОУ."кодирование ОС" ("Режимы машины состояний ОУ")) -> (s? t:f=w561:T1)
      }
      frame "отправка ОС" {
        n312 = Array Size(array=w577) -> (size(s)=w583:i32)
        n313 = call "Counter (SubVI).vi"("Counter End  Value"=u32 6) -> ("End Reached"=w582:bool)  [unwired: 9 in, 1 out]
        n314 = To Unsigned Long Integer(number=w583) -> (unsigned 32bit integer=w584:u32)
        n315 = call "Counter (SubVI).vi"("Input Valid"=w582, "Counter End  Value"=w584) -> ("Counter Value"=w578:u32, "End Reached"=w573:bool)  [unwired: 8 in]
        n316 = To Long Integer(number=w578) -> (32bit integer=w580:i32)
        n317 = Index Array(array=w577, index=w580) -> (element=w579:bool)
        n318 = local write "TX"(w579) -> ()
        n319 = case shown="True" w573 {
          frame False {
          }
          frame True {
            n320 = local write "TX"(FALSE ("TX")) -> ()
          }
        }
        n321 = local read "Передача данных\n на ОУ?"() -> (w587:bool)
        n322 = Select(t=машина_состояний_ОУ."ожидание rising" ("Режимы машины состояний ОУ"), s=w587, f=машина_состояний_ОУ."подготовка СД" ("Режимы машины состояний ОУ")) -> (s? t:f=w576:T1)
        n323 = Select(t=w576, s=w573, f=машина_состояний_ОУ."отправка ОС" ("Режимы машины состояний ОУ")) -> (s? t:f=w574:T1)
      }
      frame "подготовка СД" {
        n324 = local read "Кол-во СД"() -> (w591:u8)
        n325 = Decrement(x=w591) -> (x-1=w590:u8)
        n326 = Index Array(array="Данные для\nотправки на КШ", index=w590) -> (element=w594:u16)
        n327 = local write "Кол-во СД"(w590) -> ()
        n328 = Number To Boolean Array(number=w594) -> (Boolean array=w593:bool[])
      }
      frame "кодирование СД" {
        n329 = call "Counter (SubVI).vi"("Counter End  Value"=u32 16) -> ("Counter Value"=w608:u32, "End Reached"=w606:bool)  [unwired: 9 in]
        n330 = To Long Integer(number=w608) -> (32bit integer=w603:i32)
        n331 = Index Array(array=w599, index=w603) -> (element=w601:bool)
        n332 = feedback #22(w598) -> (w602:bool)
        n333 = Exclusive Or(1:w602, 2:w601) -> (0:w600:bool)
        n334 = feedback-in #22(w600) -> ()
        n335 = Select(t=bool[] [TRUE, FALSE], s=w601, f=bool[] [FALSE, TRUE]) -> (s? t:f=w609:bool[])
        n336 = Insert Into Array(array=w610, new element=w609) -> (w605:bool[])  [unwired: 1 in]
        n337 = case shown="True" w606 {
          tunnel: w605 -> [w614 w620]
          tunnel: [w614 w621] -> w604
          tunnel: w600 -> [_ w617]
          frame False {
          }
          frame True {
            n338 = case shown="False" w617 {
              tunnel: [bool[] [FALSE, TRUE] bool[] [TRUE, FALSE]] -> w616
              frame False {
              }
              frame True {
              }
            }
            n339 = Insert Into Array(array=w620, index=32, new element=w616) -> (w619:bool[])
            n340 = Insert Into Array(array=w619, index=0, new element=bool[] [FALSE, FALSE, FALSE, FALSE, TRUE, TRUE, TRUE]) -> (w621:bool[])
          }
        }
        n341 = Select(t=машина_состояний_ОУ."отправка СД" ("Режимы машины состояний ОУ"), s=w606, f=машина_состояний_ОУ."кодирование СД" ("Режимы машины состояний ОУ")) -> (s? t:f=w613:T1)
      }
      frame "отправка СД" {
        n342 = flat-sequence {
          tunnel: w630 -> [w631]
          frame #0 {
            n343 = for {
              tunnel: w631 -> [w633] mode=indexing
              n344 = Wait Until Next ms Multiple(millisecond multiple=u32 60) -> ()  [unwired: 1 out]
              n345 = local write "TX"(w633) -> ()
            }
          }
          frame #1 {
            n346 = local write "TX"(FALSE ("TX")) -> ()
          }
        }
        n347 = local read "Кол-во СД"() -> (w627:u8)
        n348 = Equal To 0?(x=w627) -> (x = 0?=w628:bool)
        n349 = Select(t=машина_состояний_ОУ."ожидание rising" ("Режимы машины состояний ОУ"), s=w628, f=машина_состояний_ОУ."подготовка СД" ("Режимы машины состояний ОУ")) -> (s? t:f=w629:T1)
      }
    }
    n350 = Wait Until Next ms Multiple(millisecond multiple=u32 10) -> ()  [unwired: 1 out]
    "Режимы машины состояний ОУ" <- w363
  }
  "TX" <- w7
